vi "FrameString.vi"(1 "Size (m)":cluster{"Width":sgl, "Height":sgl}, 2 "Center coordinates (m)":cluster{"Xc":sgl, "Yc":sgl}) -> (0 "string":string)   [LabVIEW 2023]
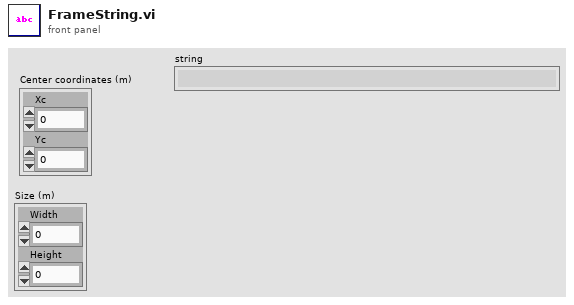
[diagram p1: front panel]
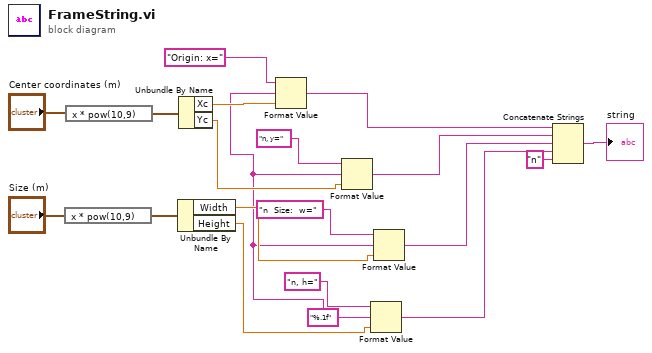
[diagram p0: block diagram]
diagram:
  w2 = "%.1f" ("format string")
  n1 = expression code="x * pow(10,9)"("Size (m)") -> (w13:cluster{"Width":sgl, "Height":sgl})
  n2 = expression code="x * pow(10,9)"("Center coordinates (m)") -> (w15:cluster{"Xc":sgl, "Yc":sgl})
  n3 = Unbundle By Name(w13) -> ("Width"=w7:sgl, "Height"=w5:sgl)
  n4 = Unbundle By Name(w15) -> ("Xc"=w18:sgl, "Yc"=w10:sgl)
  n5 = Format Value(string ("")="Origin: x=" ("string"), format string=w2, value (0)=w18) -> (output string=w12:string)
  n6 = Format Value(string ("")="n, y=" ("string"), format string=w2, value (0)=w10) -> (output string=w9:string)
  n7 = Format Value(string ("")="n, h=" ("string"), format string=w2, value (0)=w5) -> (output string=w3:string)
  n8 = Format Value(string ("")="n  Size:  w=" ("string"), format string=w2, value (0)=w7) -> (output string=w4:string)
  n9 = Concatenate Strings(w12, w9, w4, w3, "n" ("string")) -> (→"string":string)
